vi "File3.vi"() -> ()   [LabVIEW 2019]
uses:
  Control 3.ctl
  Control 1.ctl
  Control 2.ctl
panel:
  out "x-1":i32
  out "size(s) 2":i32
  in  "Rychlost ubihani":T1=0.1 step=5e-05
  out "XY Graph":cluster{dbl[], dbl[]}(graph)
  in  "stop":bool
  out "size(s)":i32
  in  "Cas necitlivosti":dbl
  out "Indexy pruchodu nulou":i32[](array[numeric])
  in  "Fvz":T2
  in  "Sirka okna (ms)":i32(listbox)
  in  "Offset":dbl format="%0.2p"
  in  "Ubihani":bool
  in  "Frekvence":dbl=10.0 format="%0.2p"
  in  "Amplituda sumu":T3
  in  "Amplituda":dbl=1.0 format="%0.2p"
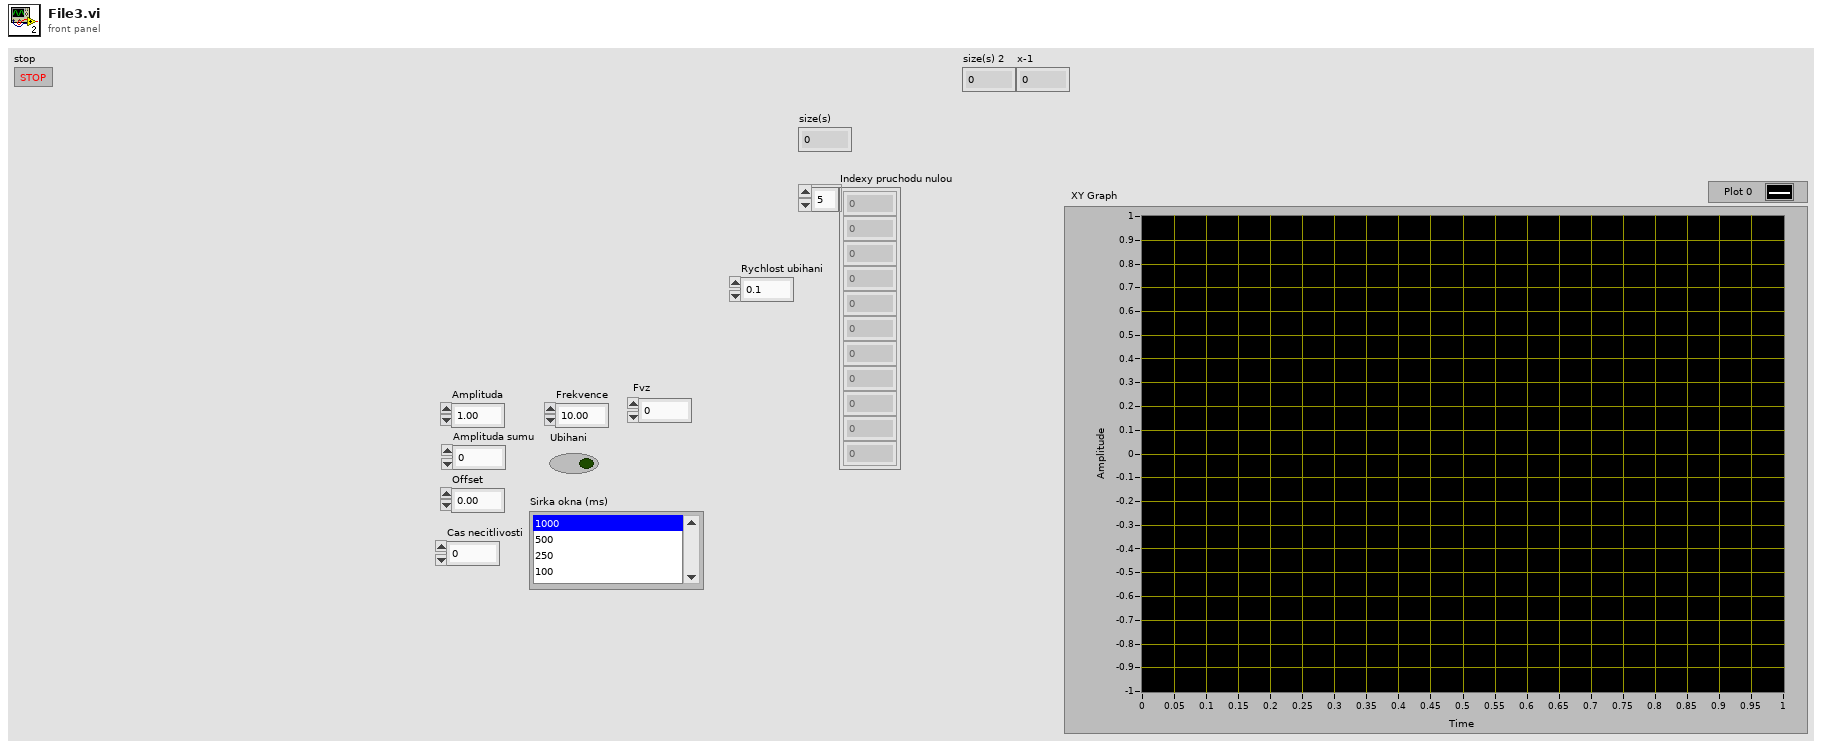
[diagram p1: front panel]
types:
  T1 = typedef "Control 2.ctl" = dbl
  T2 = typedef "Control 1.ctl" = dbl
  T3 = typedef "Control 3.ctl" = dbl
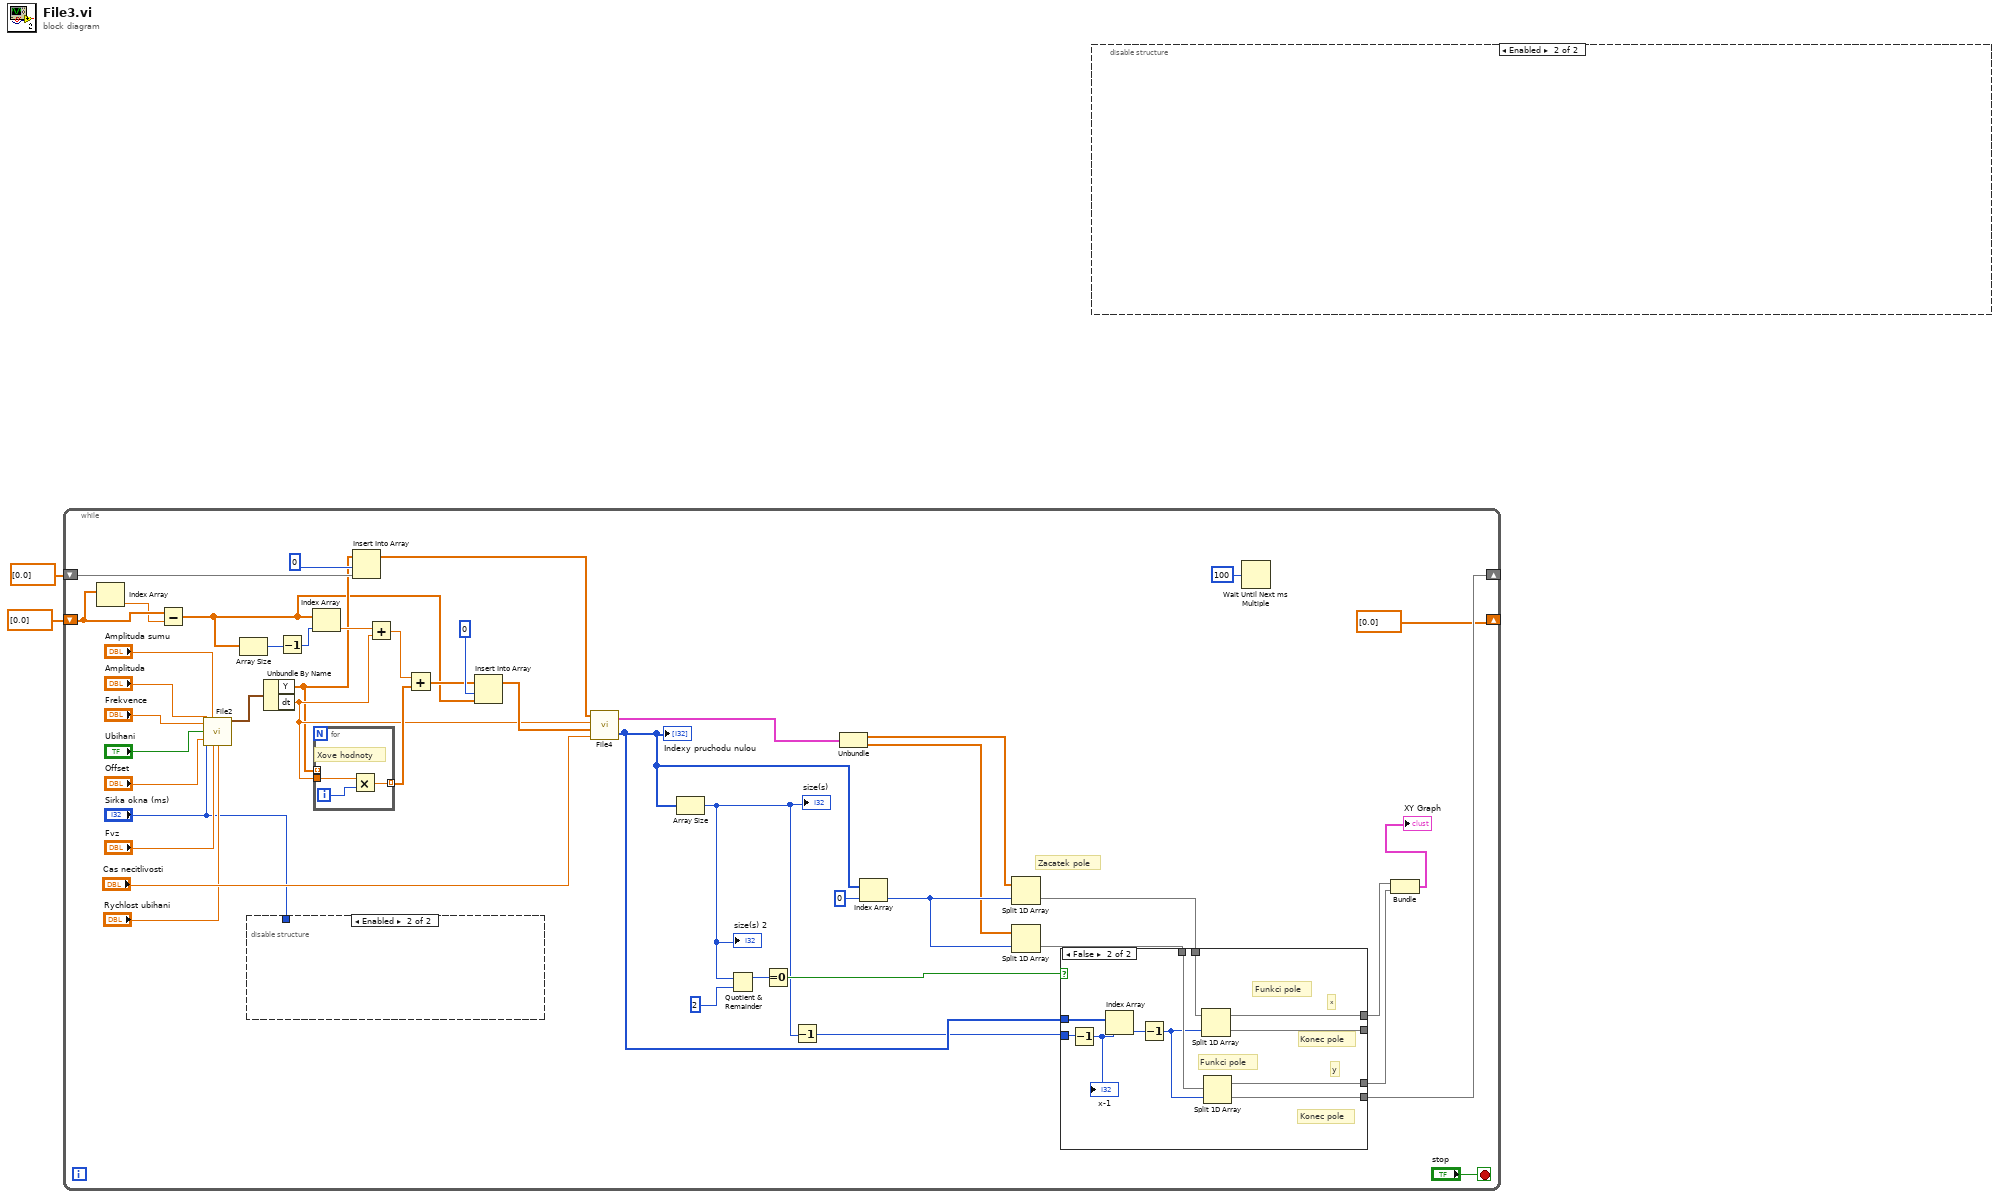
[diagram p0: block diagram]
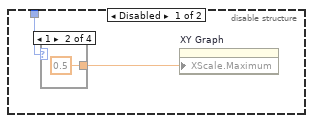
[diagram p2: hidden frame]
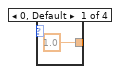
[diagram p3: hidden frame]
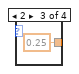
[diagram p4: hidden frame]
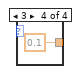
[diagram p5: hidden frame]
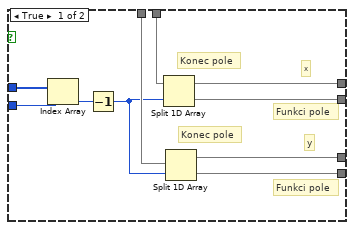
[diagram p6: hidden frame]
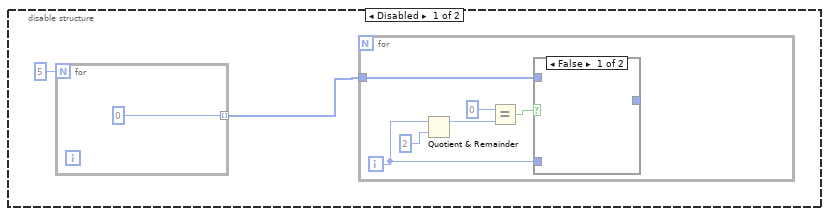
[diagram p7: hidden frame]
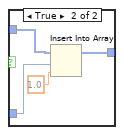
[diagram p8: hidden frame]
diagram:
  n1 = while {
    shift-right: [w10] -> _
    shift-left: dbl[] [0.0] -> [w26]
    shift-right: [dbl[] [0.0]] -> _
    shift-left: dbl[] [0.0] -> [w25]
    stop <- "stop" stop-if-true
    # "Zacatek pole"
    n2 = Index Array(array=w25) -> (element=w24:dbl)  [unwired: 1 in]
    n3 = Subtract(x=w25, y=w24) -> (x-y=w13:dbl[])
    n4 = call "File2.vi"("Amplituda"="Amplituda", "Amplituda sumu"="Amplituda sumu", "Rychlost ubihani"="Rychlost ubihani", "Frekvence"="Frekvence", "Ubihani"="Ubihani", "Offset"="Offset", "Pocet vzorku"="Sirka okna (ms)", "Fvz"="Fvz") -> ("Output"=w29:waveform(dbl))  [unwired: 6 in, 1 out]
    n5 = Array Size(array=w13) -> (size(s)=w23:i32)
    n6 = disable-structure shown="Enabled" {
      disable-tunnel: "Sirka okna (ms)" -> [w50 _]
      frame Disabled {
        n7 = case shown="1" w50 {
          tunnel: [1.0 ("X Scale.Range:Maximum") 0.5 ("X Scale.Range:Maximum") 0.25 ("X Scale.Range:Maximum") 0.1 ("X Scale.Range:Maximum")] -> w49
          frame 0, Default {
          }
          frame 1 {
          }
          frame 2 {
          }
          frame 3 {
          }
        }
        n8 = property on="XY Graph" class="XYGraph (strict)"("XScale.Maximum"=w49) -> ()  [unwired: 2 in, 2 out]
      }
      frame Enabled {
      }
    }
    n9 = Unbundle By Name(w29) -> ("Y"=w14:dbl[], "dt"=w15:dbl)
    n10 = Decrement(x=w23) -> (x-1=w22:i32)
    n11 = Index Array(array=w13, index=w22) -> (element=w21:dbl)
    n12 = for {
      tunnel: w15 -> [w57]
      tunnel: [w55] -> w18 mode=indexing
      tunnel: w14 -> [_] mode=indexing
      i -> [w56]
      # "Xove hodnoty"
      n13 = Multiply(x=w57, y=w56) -> (x*y=w55:dbl)
    }
    n14 = Insert Into Array(array=w14, index=0, new element=w26) -> (w16:dbl[])
    n15 = Add(x=w21, y=w15) -> (x+y=w20:dbl)
    n16 = Add(x=w20, y=w18) -> (x+y=w19:dbl[])
    n17 = Insert Into Array(array=w19, index=0, new element=w13) -> (w17:dbl[])
    n18 = call "File4.vi"("Pocet ignorovanych vzorku"="Cas necitlivosti", "X"=w17, "dt"=w15, "Y"=w16) -> ("Indexy pruchodu nulou"=w7:i32[], "XY Graph"=w28:cluster{"Array":dbl[], "Y":dbl[]})
    "Indexy pruchodu nulou" <- w7
    n19 = Array Size(array=w7) -> (size(s)=w38:i32)
    "size(s)" <- w38
    "size(s) 2" <- w38
    n20 = Quotient & Remainder(x=w38, y=2) -> (x-y*floor(x/y)=w40:i32)  [unwired: 1 out]
    n21 = Equal To 0?(x=w40) -> (x = 0?=w39:bool)
    n22 = Decrement(x=w38) -> (x-1=w6:i32)
    n23 = Unbundle(w28) -> ("Array"=w30:dbl[], "Y"=w31:dbl[])
    n24 = Index Array(array=w7, index=0) -> (element=w36:i32)
    n25 = Split 1D Array(array=w30, index=w36) -> (second subarray=w37:dbl[])  [unwired: 1 out]
    n26 = Split 1D Array(array=w31, index=w36) -> (second subarray=w35:dbl[])  [unwired: 1 out]
    n27 = case shown="False" w39 {
      tunnel: w37 -> [w67 w78]
      tunnel: [w66 w77] -> _
      tunnel: w35 -> [w65 w76]
      tunnel: [w64 w75] -> w10
      tunnel: [w63 w74] -> w9
      tunnel: [w62 w73] -> w11
      tunnel: w7 -> [w61 w71]
      tunnel: w6 -> [w60 w69]
      frame True {
        # "y"
        # "x"
        # "Funkci pole"
        # "Konec pole"
        # "Funkci pole"
        # "Konec pole"
        n28 = Index Array(array=w61, index=w60) -> (element=w59:i32)
        n29 = Decrement(x=w59) -> (x-1=w58:i32)
        n30 = Split 1D Array(array=w67, index=w58) -> (first subarray=w62:dbl[], second subarray=w66:dbl[])
        n31 = Split 1D Array(array=w65, index=w58) -> (first subarray=w63:dbl[], second subarray=w64:dbl[])
      }
      frame False {
        # "y"
        # "x"
        # "Funkci pole"
        # "Konec pole"
        # "Funkci pole"
        # "Konec pole"
        n32 = Decrement(x=w69) -> (x-1=w68:i32)
        "x-1" <- w68
        n33 = Index Array(array=w71, index=w68) -> (element=w70:i32)
        n34 = Decrement(x=w70) -> (x-1=w72:i32)
        n35 = Split 1D Array(array=w78, index=w72) -> (first subarray=w73:dbl[], second subarray=w77:dbl[])
        n36 = Split 1D Array(array=w76, index=w72) -> (first subarray=w74:dbl[], second subarray=w75:dbl[])
      }
    }
    n37 = Wait Until Next ms Multiple(millisecond multiple=u32 100) -> ()  [unwired: 1 out]
    n38 = Bundle(w11, w9) -> (→"XY Graph":cluster{dbl[], dbl[]})  [unwired: 1 in]
  }
  n39 = disable-structure shown="Enabled" {
    frame Disabled {
      n40 = for {
        N: 5 -> [_]
        tunnel: [0] -> w79 mode=indexing
      }
      n41 = for {
        tunnel: w79 -> [w81]
        i -> [w82]
        n42 = Quotient & Remainder(x=w82, y=2) -> (x-y*floor(x/y)=w85:i32)  [unwired: 1 out]
        n43 = Equal?(x=0, y=w85) -> (x = y?=w83:bool)
        n44 = case shown="False" w83 {
          tunnel: w82 -> [_ w90]
          tunnel: w81 -> [_ w88]
          tunnel: [_ w87] -> _
          frame False {
          }
          frame True {
            n45 = Insert Into Array(array=w88, index=w90, new element=1.0 ("new element/subarray")) -> (w87:i32[])
          }
        }
      }
    }
    frame Enabled {
    }
  }
